vi "T Gate.vi"(2 "v Ctrl in":refnum<class "CtrlLine.lvclass">, 7 "QuWire in":refnum<class "QuWire.lvclass">, 13 "^ Ctrl in":refnum<class "CtrlLine.lvclass">) -> (8 "QuWire out":refnum<class "QuWire.lvclass">)   [LabVIEW 2020]
doc: "T Gate (pi/8)\n\nApplies a pi/4 phase shift. \nT = sqrt(S). \nMaps |1> to e^(ipi/4)|1>. \n\nMatrix: [[ 1, 0], [ 0, exp(i*pi/4) ]]"
uses:
  QuSim/QuWire/QuWire.lvclass
  QuSim/QuWire/CtrlLine/CtrlLine.lvclass
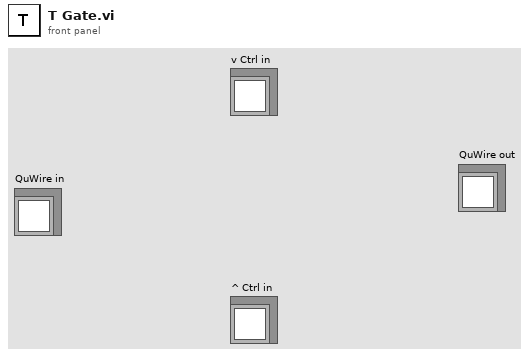
[diagram p1: front panel]
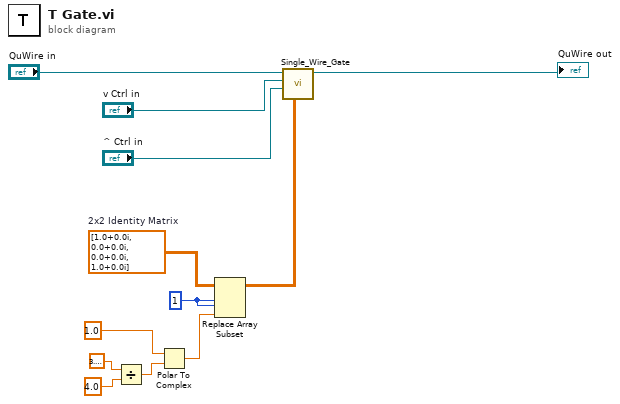
[diagram p0: block diagram]
diagram:
  w7 = 1 ("index (row)")
  w8 = cdb[][] [[1.0+0.0i, 0.0+0.0i], [0.0+0.0i, 1.0+0.0i]]  # 2x2 Identity Matrix
  n1 = Divide(x=3.141592653589793 ("Pi"), y=4.0) -> (x/y=w3:dbl)
  n2 = Polar To Complex(1:w3, 2:1.0 ("r")) -> (0:w1:cdb)
  n3 = Replace Array Subset(array=w8, new element=w1, index (row)=w7, index (col)=w7) -> (w6:cdb[][])
  n4 = call "Single_Wire_Gate.vi"("2x2 Unitary Matrix"=w6, "d CtrlLine in"="^ Ctrl in", "u CtrlLine in"="v Ctrl in", "QuWire in"="QuWire in") -> ("QuWire out"=→"QuWire out":refnum<class "QuWire.lvclass">)  [unwired: 6 in, 1 out]
